vi "test_Error Code and Message Status Channels by Generating Protection Error (-265).vi"(8 "error in (no error)":errorcluster, 11 "TestCase in":refnum<class "Instrument Addon Error System Tests.lvclass">) -> (0 "error out":errorcluster, 3 "TestCase out":refnum<class "Instrument Addon Error System Tests.lvclass">)   [LabVIEW 2019, in "Instrument Addon Error System Tests.lvclass"]
uses:
  Instrument Addon Error System Tests.lvclass
  C:/Program Files (x86)/National Instruments/LabVIEW 2019/vi.lib/NI/VeriStand Custom Device Testing Tools/VeriStandTestCase/VeriStandTestCase.lvclass
  <vilib>/NI VeriStand/Execution/Workspace/NI VeriStand - Set Multiple Channel Values.vi
  <vilib>/NI VeriStand/Execution/Workspace/NI VeriStand - Get Multiple Channel Values.vi
  <vilib>/addons/_JKI Toolkits/VI Tester/TestCase.llb/TestCase.lvclass
  <vilib>/NI VeriStand/Execution/Workspace/NI_VS Workspace ExecutionAPI.lvlib
  C:/Program Files (x86)/National Instruments/LabVIEW 2019/vi.lib/addons/_JKI Toolkits/VI Tester/TestCase.llb/TestCase.lvclass
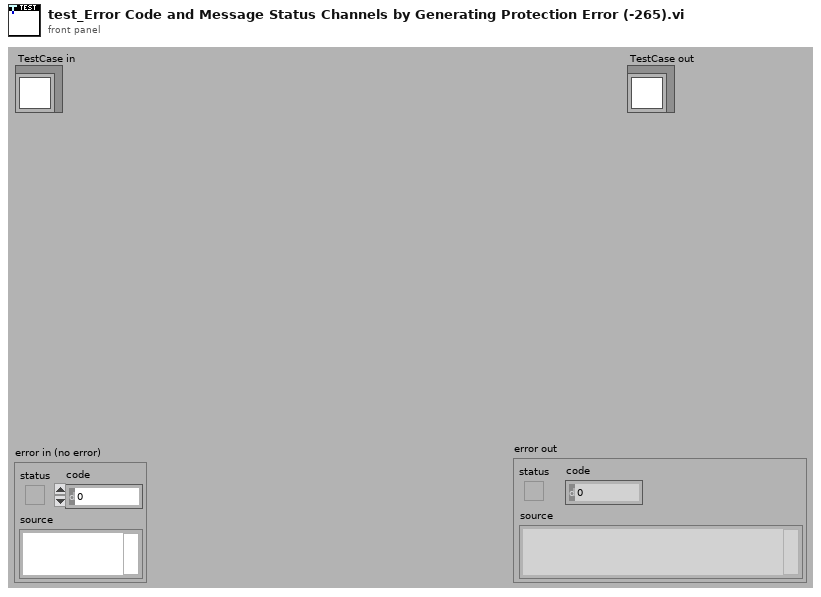
[diagram p1: front panel]
types:
  T1 = typedef "NI_VS Workspace ExecutionAPI.lvlib/WorkspaceAPI.ctl" = refnum<k24>
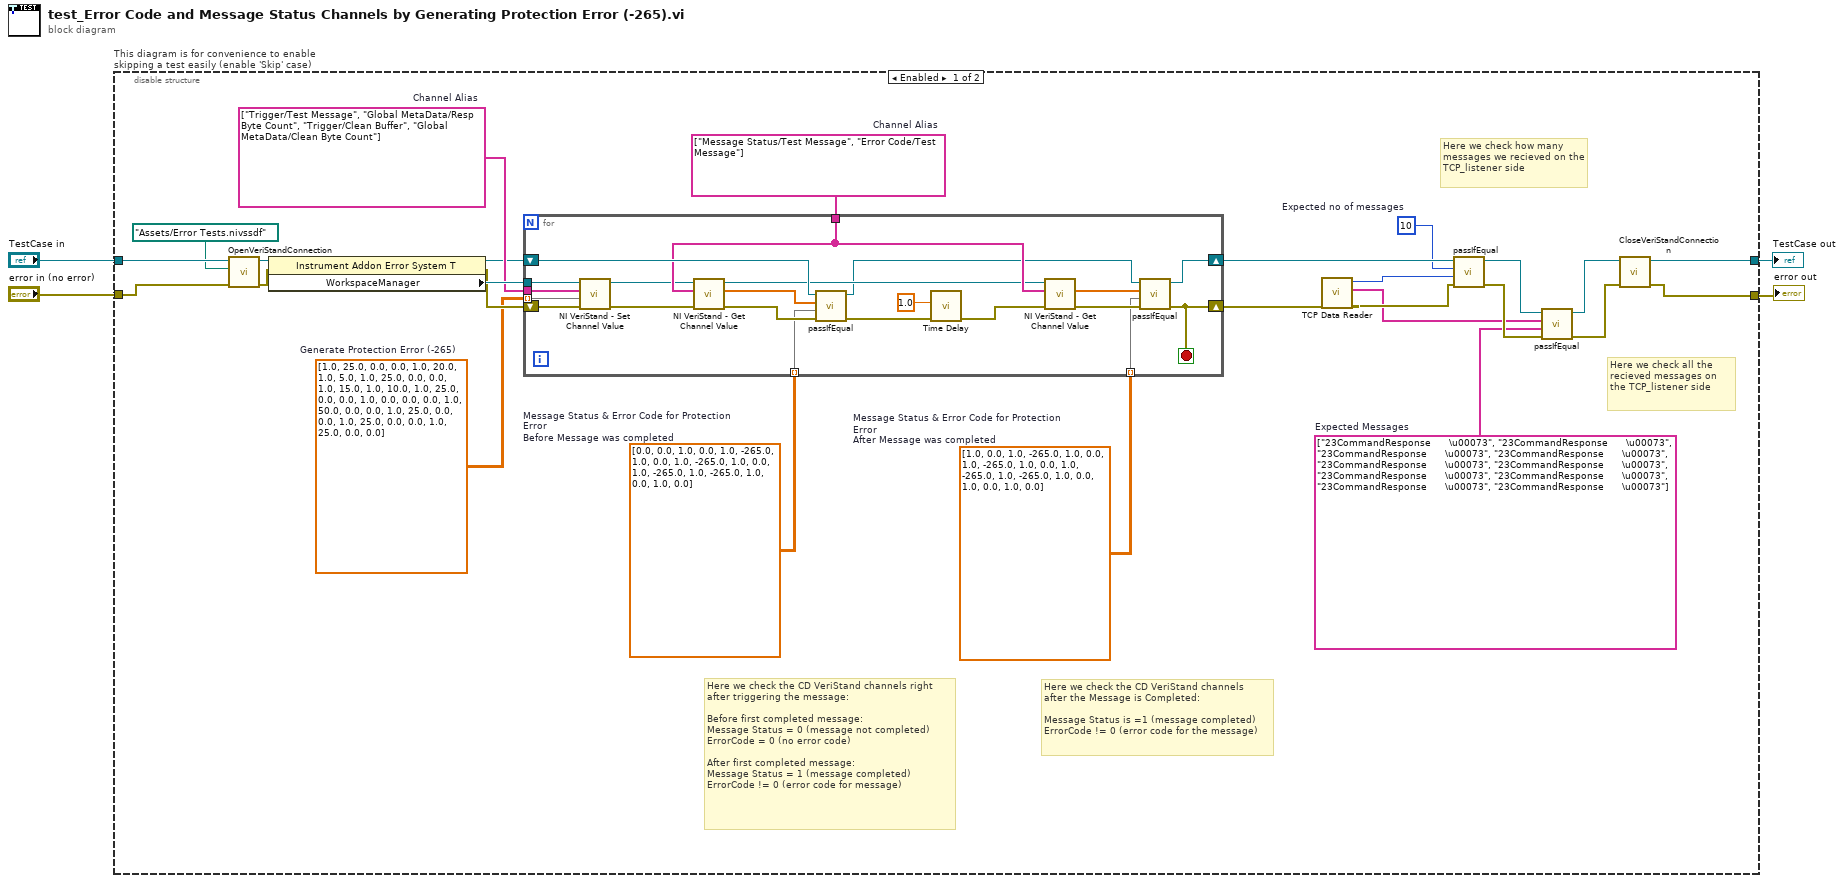
[diagram p0: block diagram]
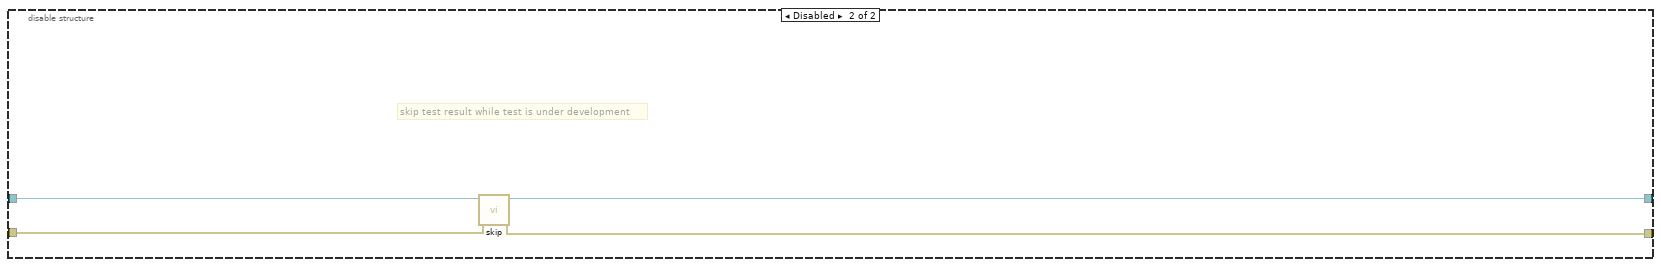
[diagram p2: hidden frame]
diagram:
  n1 = disable-structure "This diagram is for convenience to enable skipping a test easily (enable 'Skip' case)" shown="Enabled" {
    disable-tunnel: "TestCase in" -> [w28 w55]
    disable-tunnel: [w29 w53] -> w1
    disable-tunnel: [w30 w54] -> w3
    disable-tunnel: "error in (no error)" -> [w26 w52]
    frame Enabled {
      w5 = dbl[][] [[1.0, 0.0], [1.0, -265.0], [1.0, 0.0], [1.0, -265.0], [1.0, 0.0], [1.0, -265.0], [1.0, -265.0], [1.0, 0.0], [1.0, 0.0], [1.0, 0.0]]  # Message Status & Error Code for Protection Error After Message was completed
      w6 = dbl[][] [[0.0, 0.0], [1.0, 0.0], [1.0, -265.0], [1.0, 0.0], [1.0, -265.0], [1.0, 0.0], [1.0, -265.0], [1.0, -265.0], [1.0, 0.0], [1.0, 0.0]]  # Message Status & Error Code for Protection Error Before Message was completed
      w7 = dbl[][] [[1.0, 25.0, 0.0, 0.0], [1.0, 20.0, 1.0, 5.0], [1.0, 25.0, 0.0, 0.0], [1.0, 15.0, 1.0, 10.0], [1.0, 25.0, 0.0, 0.0], [1.0, 0.0, 0.0, 0.0], [1.0, 50.0, 0.0, 0.0], [1.0, 25.0, 0.0, 0.0], [1.0, 25.0, 0.0, 0.0], [1.0, 25.0, 0.0, 0.0]]  # Generate Protection Error (-265)
      w14 = string[] ["23CommandResponse      \u00073", "23CommandResponse      \u00073", "23CommandResponse      \u00073", "23CommandResponse      \u00073", "23CommandResponse      \u00073", "23CommandResponse      \u00073", "23CommandResponse      \u00073", "23CommandResponse      \u00073", "23CommandResponse      \u00073", "23CommandResponse      \u00073"]  # Expected Messages
      w8 = string[] ["Message Status/Test Message", "Error Code/Test Message"]  # Channel Alias
      w13 = 10  # Expected no of messages
      w21 = string[] ["Trigger/Test Message", "Global MetaData/Resp Byte Count", "Trigger/Clean Buffer", "Global MetaData/Clean Byte Count"]  # Channel Alias
      # "Here we check the CD VeriStand channels right\nafter triggering the message:\n\nBefore first completed message:\nMessage Status = 0 (message not completed)\nErrorCode = 0 (no error code)\n\nAfter first completed message:\nMessage Status = 1 (message completed)\nErrorCode != 0 (error code for message)"
      # "Here we check all the recieved messages on the TCP_listener side"
      # "Here we check how many messages we recieved on the TCP_listener side"
      # "Here we check the CD VeriStand channels\nafter the Message is Completed:\n\nMessage Status is =1 (message completed)\nErrorCode != 0 (error code for the message)"
      n2 = call-dynamic "OpenVeriStandConnection.vi"("error in (no error)"=w26, "System Definition File"=path "Assets/Error Tests.nivssdf", "VeriStand Test Case in"=w28) -> ("error out"=w25:errorcluster, "VeriStand Test Case out"=w27:refnum<class "Instrument Addon Error System Tests.lvclass">)  [unwired: 6 in, 1 out]
      n3 = property class="Instrument Addon Error System T"(reference=w27, error in=w25) -> (reference out=w20:refnum<class "Instrument Addon Error System Tests.lvclass">, error out=w22:errorcluster, "WorkspaceManager"=w23:T1)
      n4 = for {
        tunnel: w23 -> [w51]
        tunnel: w21 -> [w49]
        tunnel: w8 -> [w46]
        tunnel: w7 -> [w45] mode=indexing
        shift-right: [w31] -> w12
        shift-left: w22 -> [w50]
        shift-right: [w47] -> w15
        shift-left: w20 -> [w48]
        tunnel: w6 -> [w34] mode=indexing
        tunnel: w5 -> [w33] mode=indexing
        stop <- w31 stop-if-true
        n5 = call-poly <vilib>:"NI VeriStand - Set Channel Value.vi"("error in (no error)"=w50, "Values"=w45, "Channels"=w49, "WorkspaceManager in"=w51) -> ("error out"=w39:errorcluster, "WorkspaceManager out"=w41:T1)  [unwired: 6 in]
        n6 = call-poly <vilib>:"NI VeriStand - Get Channel Value.vi"("error in (no error)"=w39, "Channels"=w46, "WorkspaceManager in"=w41) -> ("error out"=w37:errorcluster, "Values"=w36:dbl[], "WorkspaceManager out"=w40:T1)  [unwired: 6 in]
        n7 = call-dynamic "passIfEqual.vi"("error in (no error)"=w37, "y"=w34, "x"=w36, "TestCase in"=w48) -> ("error out"=w32:errorcluster, "TestCase out"=w38:refnum<class "Instrument Addon Error System Tests.lvclass">)  [unwired: 6 in]
        n8 = call "Time Delay"("error in (no error)"=w32, "Delay Time (s)"=1.0) -> ("error out"=w43:errorcluster)  [unwired: 9 in]
        n9 = call-poly <vilib>:"NI VeriStand - Get Channel Value.vi"("error in (no error)"=w43, "Channels"=w46, "WorkspaceManager in"=w40) -> ("error out"=w42:errorcluster, "Values"=w35:dbl[])  [unwired: 6 in, 1 out]
        n10 = call-dynamic "passIfEqual.vi"("error in (no error)"=w42, "y"=w33, "x"=w35, "TestCase in"=w38) -> ("error out"=w31:errorcluster, "TestCase out"=w47:refnum<class "Instrument Addon Error System Tests.lvclass">)  [unwired: 6 in]
      }
      n11 = call "TCP Data Reader.vi"("error in (no error)"=w12) -> ("error out"=w10:errorcluster, "Recieved Messages"=w9:string[], "No of messages"=w11:i32)  [unwired: 8 in]
      n12 = call-dynamic "passIfEqual.vi"("error in (no error)"=w10, "y"=w11, "x"=w13, "TestCase in"=w15) -> ("error out"=w17:errorcluster, "TestCase out"=w19:refnum<class "Instrument Addon Error System Tests.lvclass">)  [unwired: 6 in]
      n13 = call-dynamic "passIfEqual.vi"("error in (no error)"=w17, "y"=w14, "x"=w9, "TestCase in"=w19) -> ("error out"=w16:errorcluster, "TestCase out"=w18:refnum<class "Instrument Addon Error System Tests.lvclass">)  [unwired: 6 in]
      n14 = call-dynamic "CloseVeriStandConnection.vi"("error in (no error)"=w16, "VeriStand Test Case in"=w18) -> ("error out"=w30:errorcluster, "VeriStand Test Case out"=w29:refnum<class "Instrument Addon Error System Tests.lvclass">)  [unwired: 8 in]
    }
    frame Disabled {
      # "skip test result while test is under development"
      n15 = call <vilib>:"skip.vi"("error in (no error)"=w52, "TestCase in"=w55) -> ("error out"=w54:errorcluster, "TestCase out"=w53:refnum<class "Instrument Addon Error System Tests.lvclass">)  [unwired: 8 in]
    }
  }
  "error out" <- w3
  "TestCase out" <- w1
